vi "point distance (in range).vi"(2 "range":T1, 3 "cartesian location":cluster{dbl, dbl}) -> (0 "distance":dbl, 1 "In Range?":bool)   [LabVIEW 2009]
panel:
  in  "polar range? (cartesian)":bool
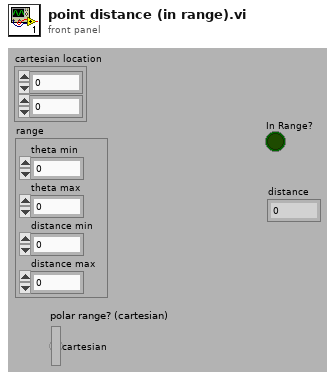
[diagram p1: front panel]
types:
  T1 = cluster{"theta min":dbl, "theta max":dbl, "distance min":dbl, "distance max":dbl}
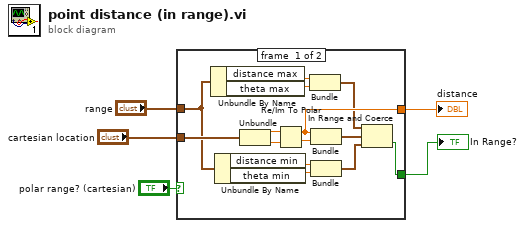
[diagram p0: block diagram]
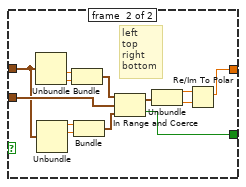
[diagram p2: hidden frame]
diagram:
  n1 = case shown="False" "polar range? (cartesian)" {
    tunnel: "cartesian location" -> [w19 w27]
    tunnel: [w16 w30] -> w4
    tunnel: "range" -> [w12 w25]
    tunnel: [w6 w29] -> w2
    frame #0 {
      n2 = Unbundle By Name(w12) -> ("distance max"=w13:dbl, "theta max"=w14:dbl)
      n3 = Unbundle By Name(w12) -> ("distance min"=w10:dbl, "theta min"=w11:dbl)
      n4 = Unbundle(w19) -> (w17:dbl, w18:dbl)
      n5 = Re/Im To Polar(2:w18, 3:w17) -> (0:w15:dbl, 1:w16:dbl)
      n6 = Bundle("distance max"=w13, "theta max"=w14) -> (w8:cluster{"distance max":dbl, "theta max":dbl})  [unwired: 1 in]
      n7 = Bundle(w16, w15) -> (w9:cluster{dbl, dbl})  [unwired: 1 in]
      n8 = Bundle("distance min"=w10, "theta min"=w11) -> (w7:cluster{"distance min":dbl, "theta min":dbl})  [unwired: 1 in]
      n9 = In Range and Coerce(upper limit=w8, x=w9, lower limit=w7) -> (In Range?=w6:bool)  [unwired: 1 out]
    }
    frame #1 {
      # "left\ntop\nright\nbottom"
      n10 = Unbundle(w25) -> ("distance min"=w23:dbl, "distance max"=w22:dbl)  [unwired: 2 out]
      n11 = Unbundle(w25) -> ("theta min"=w21:dbl, "theta max"=w20:dbl)  [unwired: 2 out]
      n12 = Bundle("distance min"=w23, "distance max"=w22) -> (w26:cluster{"distance min":dbl, "distance max":dbl})  [unwired: 1 in]
      n13 = Bundle("theta min"=w21, "theta max"=w20) -> (w24:cluster{"theta min":dbl, "theta max":dbl})  [unwired: 1 in]
      n14 = In Range and Coerce(upper limit=w26, x=w27, lower limit=w24) -> (coerced(x)=w28:cluster{"distance min":dbl, "distance max":dbl}, In Range?=w29:bool)
      n15 = Unbundle(w28) -> ("distance min"=w31:dbl, "distance max"=w32:dbl)
      n16 = Re/Im To Polar(2:w32, 3:w31) -> (1:w30:dbl)  [unwired: 1 out]
    }
  }
  "distance" <- w4
  "In Range?" <- w2
